vi "DxfRead.vi"(8 "error in (no error)":errorcluster) -> (0 "error out":errorcluster, 1 "Array 2":T1[](array[typedef]), 2 "Array":cluster{string, dbl[]}[](array[cluster]), 3 "stripped path":path, 5 "name":string)   [LabVIEW 2018]
uses:
  typeDefs/singleDXFobject.ctl
  typeDefs/singleDXFvar.ctl
  Dxf.lvlib
  dxf typedef.lvlib
panel:
  # "Connector Pane"
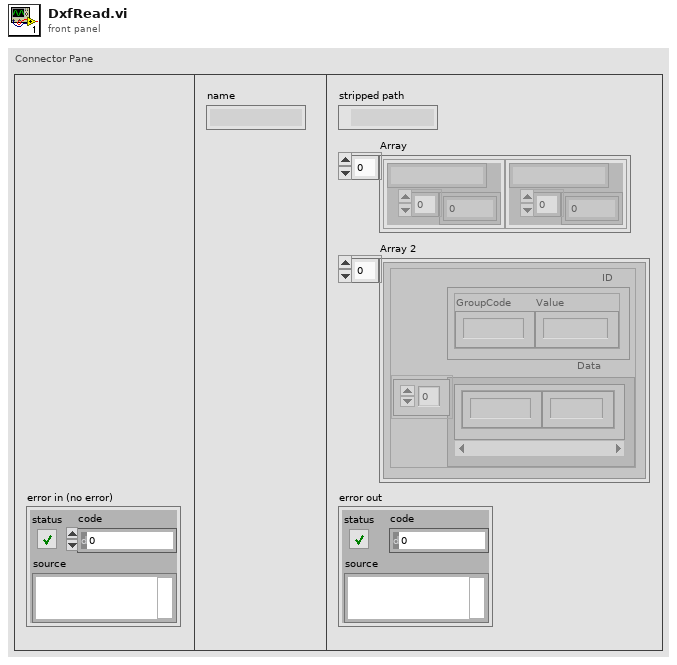
[diagram p1: front panel]
types:
  T1 = typedef "dxf typedef.lvlib/singleDXFobject.ctl" = cluster{"ID":T2, "Data":T2[]}
  T2 = typedef "dxf typedef.lvlib/singleDXFvar.ctl" = cluster{"GroupCode":string, "Value":string}
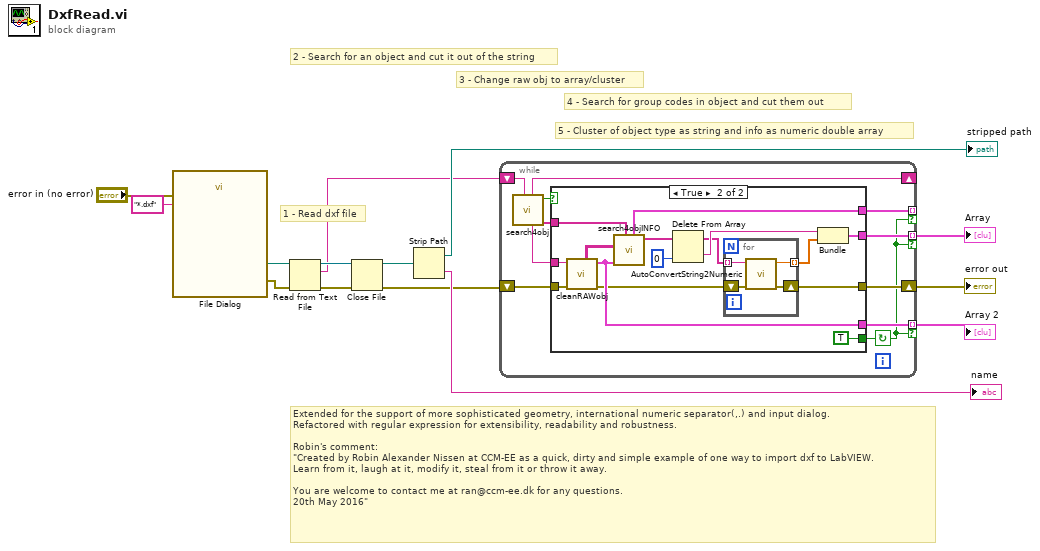
[diagram p0: block diagram]
diagram:
  # "Extended for the support of more sophisticated geometry, international numeric separator(,.) and input dialog.\nRefactored with regular expression for extensibility, readability and robustness.\n\nRobin's comment: \n\"Created by Robin Alexander Nissen at CCM-EE as a quick, dirty and simple example of one way to import dxf to LabVIEW.\nLearn from it, laugh at it, modify it, steal from it or throw it away.\n\nYou are welcome to contact me at ran@ccm-ee.dk for any questions.\n20th May 2016\""
  # "5 - Cluster of object type as string and info as numeric double array"
  # "4 - Search for group codes in object and cut them out"
  # "3 - Change raw obj to array/cluster"
  # "1 - Read dxf file"
  # "2 - Search for an object and cut it out of the string"
  n1 = call "File Dialog"("error in"="error in (no error)", "pattern (all files)"="*.dxf") -> ("selected path"=w4:path, "error out"=w3:errorcluster)  [unwired: 10 in, 2 out]
  n2 = Read from Text File(file (use dialog)=w4, error in=w3) -> (refnum out=w6:refnum<file>, text=w5:string, error out=w7:errorcluster)  [unwired: 2 in, 1 out]
  n3 = Close File(refnum=w6, error in=w7) -> (path=w10:path, error out=w8:errorcluster)
  n4 = Strip Path(path=w10) -> (stripped path=→"stripped path":path, name=→"name":string)
  n5 = while {
    shift-right: [w17] -> _
    shift-left: w5 -> [w18]
    tunnel: [w21] -> w9 mode=indexing if=w16
    tunnel: [w25] -> w11 mode=indexing if=w16
    shift-right: [w23] -> w14
    shift-left: w8 -> [w24]
    tunnel: [w15] -> _ mode=indexing if=w16
    stop <- w16 continue-if-true
    n6 = call "search4obj.vi"("raw dxf in"=w18) -> ("deafult obj properies of interest"=w20:string[], "obj found?"=w19:bool, "found dxf obj raw"=w22:string, "raw dxf minus object found"=w17:string)  [unwired: 7 in]
    n7 = case shown="True" w19 {
      tunnel: [_ w41] -> w25
      tunnel: w24 -> [w26 w28]
      tunnel: [w26 w40] -> w23
      tunnel: w22 -> [_ w31]
      tunnel: [_ w29] -> w21
      tunnel: w20 -> [_ w39]
      tunnel: [_ TRUE] -> w16
      tunnel: [_ w32] -> w15
      frame False {
      }
      frame True {
        n8 = call "cleanRAWobj.vi"("error in (no error)"=w28, "raw dxf obj in"=w31) -> ("error out"=w27:errorcluster, "dxfObject"=w29:T1, "complete obj as 2Darray out"=w30:string[][])  [unwired: 7 in]
        n9 = call "search4objINFO.vi"("obj properties of interest"=w39, "dxfObject in"=w29, "complete obj in"=w30) -> ("obj of interest data out"=w34:string[], "dxfObject of interest out"=w32:T1)  [unwired: 7 in]
        n10 = Delete From Array(array=w34, index=0) -> (deleted portion=w36:string, array with subset deleted=w35:string[])  [unwired: 1 in]
        n11 = for {
          tunnel: w35 -> [w45] mode=indexing
          tunnel: [w42] -> w37 mode=indexing
          shift-right: [w43] -> w40
          shift-left: w27 -> [w44]
          n12 = call "AutoConvertString2Numeric.vi"("error in (no error)"=w44, "string in"=w45) -> ("error out"=w43:errorcluster, "Numeric out"=w42:dbl)  [unwired: 8 in]
        }
        n13 = Bundle(w36, w37) -> (w41:cluster{string, dbl[]})  [unwired: 1 in]
      }
    }
  }
  "error out" <- w14
  "Array" <- w11
  "Array 2" <- w9
